vi "Create.vi"(8 "error in (no error)":errorcluster, 10 "String":string) -> (0 "error out":errorcluster, 3 "Descrambler":refnum<class "Descrambler.lvclass">)   [LabVIEW 2020, in "Descrambler.lvclass"]
uses:
  Descrambler.lvclass
  Descrambler.lvclass/Descrambler.ctl
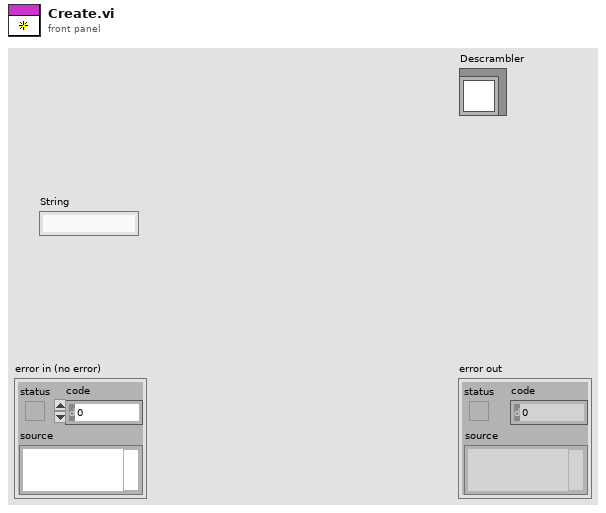
[diagram p1: front panel]
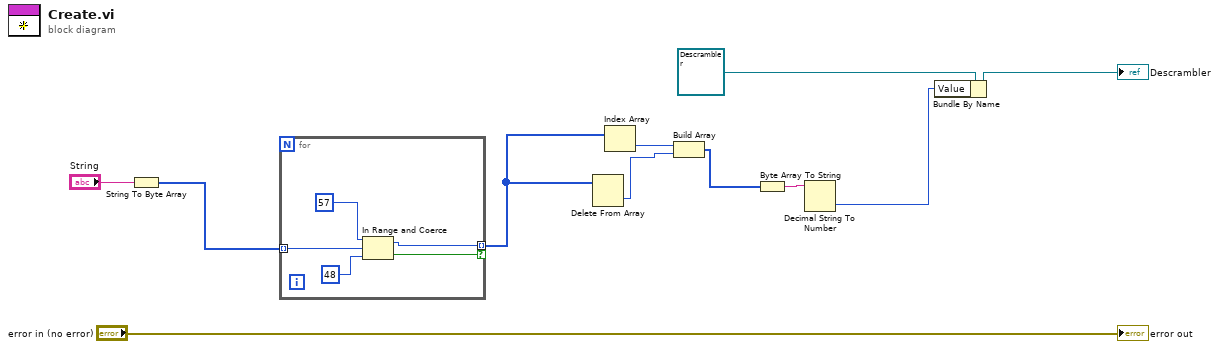
[diagram p0: block diagram]
diagram:
  n1 = String To Byte Array(string="String") -> (unsigned byte array=w8:u8[])
  n2 = for {
    tunnel: w8 -> [w16] mode=indexing
    tunnel: [w15] -> w4 mode=indexing if=w12
    n3 = In Range and Coerce(upper limit=57, x=w16, lower limit=48) -> (coerced(x)=w15:i32, In Range?=w12:bool)
  }
  n4 = Delete From Array(array=w4) -> (deleted portion=w2:i32)  [unwired: 2 in, 1 out]
  n5 = Index Array(array=w4) -> (element=w3:i32)  [unwired: 1 in]
  n6 = Build Array(w3, w2) -> (w1:i32[])
  n7 = Byte Array To String(unsigned byte array=w1) -> (string=w7:string)
  n8 = Decimal String To Number(string=w7) -> (number=w5:i32)  [unwired: 2 in, 1 out]
  n9 = Bundle By Name(cluster=refnum<class "Descrambler.lvclass"> refnum ("Descrambler"), "Value"=w5) -> (→"Descrambler":refnum<class "Descrambler.lvclass">)
  "error out" <- "error in (no error)"
